vi "OCR_Build Lookup arrays.vi"(8 "Error":errorcluster) -> (0 "Error Out":errorcluster, 3 "Look Up Array Out":cluster{T1[]}[](array[cluster]))   [LabVIEW 2009]
doc: "Builds Lookup arrays from font list"
uses:
  Controls/Cluster/Cluster_Bit array and Character.ctl
  Controls/Array/Array Bool Char Bits Wide.ctl
  Controls/String_Picture/String Char Normal.ctl
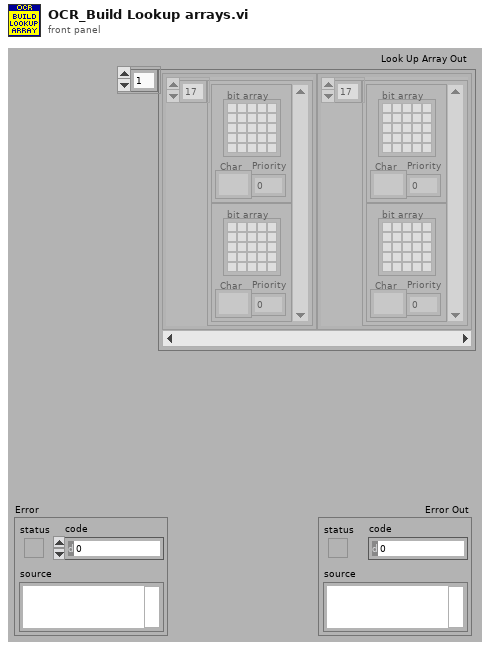
[diagram p1: front panel]
types:
  T1 = typedef "Cluster_Bit array and Character.ctl" = cluster{"bit array":T2, "Char":T3, "Priority":i32}
  T2 = typedef "Array Bool Char Bits Wide.ctl" = bool[][]
  T3 = typedef "String Char Normal.ctl" = string
  T4 = typedef "Cluster_Font Data.ctl" = cluster{"Font List Out":T5[], "Char Array":T3[], "Seperator Index":i32}
  T5 = typedef "Cluster_Character Data.ctl" = cluster{"Char":T3, "Wide":T2, "Med":T6, "Thin":T7, "Priority":i32}
  T6 = typedef "Array Bool Char Bits Med.ctl" = bool[][]
  T7 = typedef "Array Bool Char Bits Thin.ctl" = bool[][]
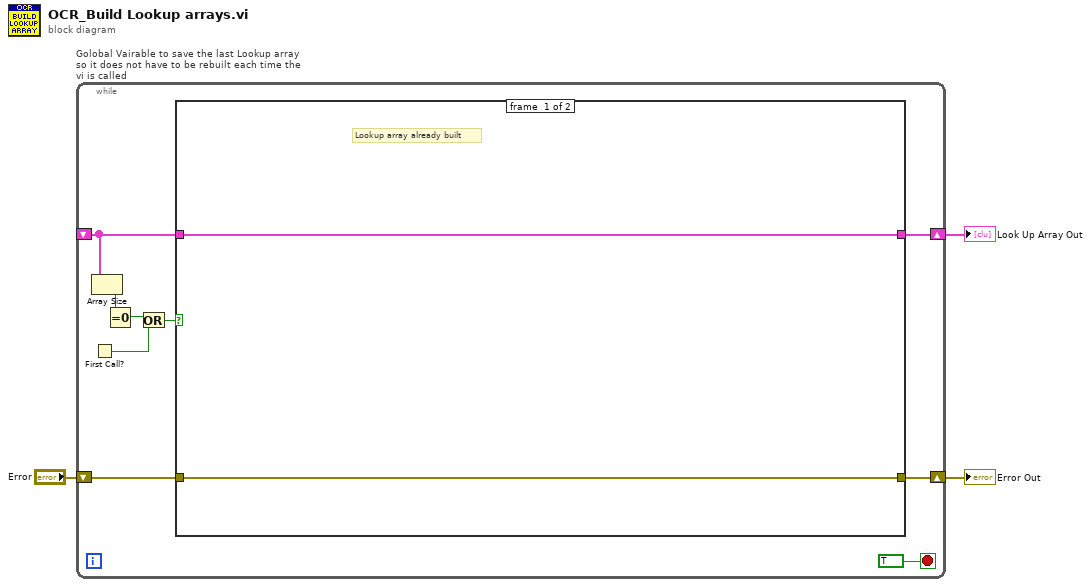
[diagram p0: block diagram]
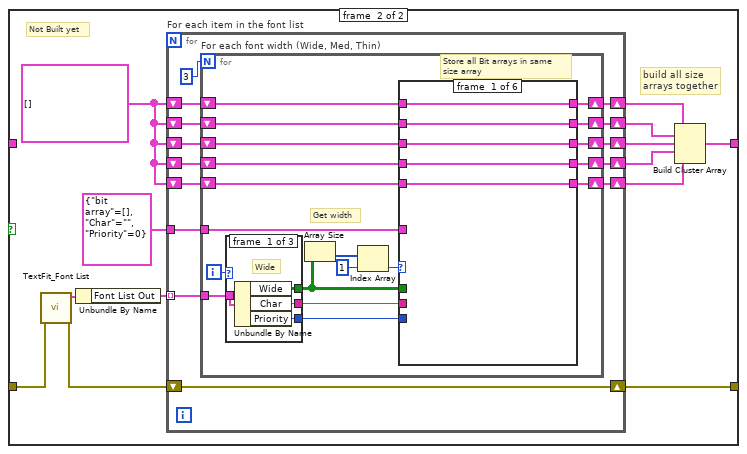
[diagram p2: hidden frame]
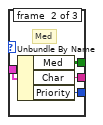
[diagram p3: hidden frame]
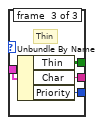
[diagram p4: hidden frame]
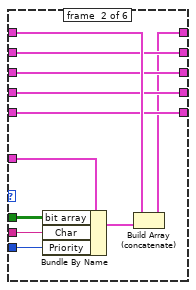
[diagram p5: hidden frame]
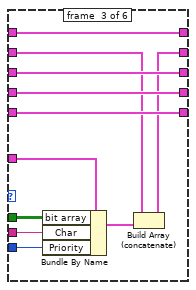
[diagram p6: hidden frame]
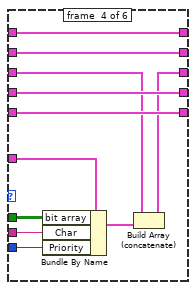
[diagram p7: hidden frame]
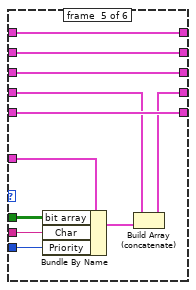
[diagram p8: hidden frame]
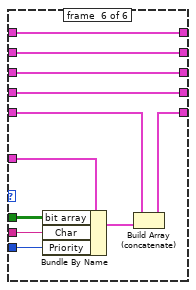
[diagram p9: hidden frame]
diagram:
  n1 = while "Golobal Vairable to save the last Lookup array so it does not have to be rebuilt each time the vi is called" {
    shift-right: [w11] -> w2
    shift-left: "Error" -> [w12]
    shift-right: [w10] -> w1
    shift-left: _ -> [w6]
    stop <- TRUE stop-if-true
    n2 = First Call?() -> (First Call?: T/F=w4:bool)
    n3 = Array Size(array=w6) -> (size(s)=w8:i32)
    n4 = Equal To 0?(x=w8) -> (x = 0?=w7:bool)
    n5 = Or(x=w7, y=w4) -> (x .or. y?=w5:bool)
    n6 = case shown="True" w5 {
      tunnel: w12 -> [w13 w27]
      tunnel: [w13 w26] -> w11
      tunnel: [w14 w15] -> w10
      tunnel: w6 -> [w14 _]
      frame #0 {
        # "Lookup array already built"
      }
      frame #1 {
        w22 = T1[] []
        # "build all size\narrays together"
        # "Not Built yet"
        n7 = call "TextFit_Font List.vi"("Error In"=w27) -> ("Error Out"=w25:errorcluster, "Font Cluster Out"=w24:T4)  [unwired: 9 in]
        n8 = Unbundle By Name(w24) -> ("Font List Out"=w23:T5[])
        n9 = for "For each item in the font list" {
          shift-right: [w41] -> w26
          shift-left: w25 -> [w41]
          tunnel: w23 -> [w38] mode=indexing
          shift-right: [w32] -> w19
          shift-left: w22 -> [w37]
          shift-right: [w31] -> w16
          shift-left: w22 -> [w36]
          shift-right: [w30] -> w20
          shift-left: w22 -> [w35]
          shift-right: [w29] -> w17
          shift-left: w22 -> [w34]
          shift-right: [w28] -> w18
          shift-left: w22 -> [w33]
          tunnel: T1 {"bit array"=[], "Char"="", "Priority"=0} ("bit char cluster") -> [w40]
          n10 = for "For each font width (Wide, Med, Thin)" {
            N: 3 -> [_]
            tunnel: w40 -> [w60]
            tunnel: w38 -> [w58]
            shift-right: [w43] -> w28
            shift-left: w33 -> [w48]
            shift-right: [w44] -> w29
            shift-left: w34 -> [w49]
            shift-right: [w45] -> w30
            shift-left: w35 -> [w50]
            shift-right: [w46] -> w31
            shift-left: w36 -> [w51]
            shift-right: [w47] -> w32
            shift-left: w37 -> [w52]
            i -> [w59]
            # "Store all Bit arrays in same\nsize array"
            # "Get width"
            n11 = case shown="..0" w59 {
              tunnel: w58 -> [w64 w68 w72]
              tunnel: [w63 w67 w71] -> w56
              tunnel: [w62 w66 w70] -> w57
              tunnel: [w61 w65 w69] -> w42
              frame #0 {
                # "Wide"
                n12 = Unbundle By Name(w64) -> ("Wide"=w63:T2, "Char"=w62:T3, "Priority"=w61:i32)
              }
              frame #1 {
                # "Med"
                n13 = Unbundle By Name(w68) -> ("Med"=w67:T6, "Char"=w66:T3, "Priority"=w65:i32)
              }
              frame #2 {
                # "Thin"
                n14 = Unbundle By Name(w72) -> ("Thin"=w71:T7, "Char"=w70:T3, "Priority"=w69:i32)
              }
            }
            n15 = Array Size(array=w56) -> (size(s)=w55:i32[])
            n16 = Index Array(array=w55, index=1) -> (element=w53:i32)
            n17 = case shown="3" w53 {
              tunnel: w60 -> [_ w83 w96 w108 w120 w132]
              tunnel: w56 -> [_ w81 w94 w106 w118 w130]
              tunnel: w57 -> [_ w82 w95 w107 w119 w131]
              tunnel: w52 -> [w77 w88 w92 w104 w116 w128]
              tunnel: w51 -> [w76 w87 w91 w101 w115 w127]
              tunnel: w50 -> [w75 w86 w99 w103 w112 w126]
              tunnel: w49 -> [w74 w85 w98 w110 w114 w123]
              tunnel: w48 -> [w73 w84 w97 w109 w121 w125]
              tunnel: [w77 w80 w92 w104 w116 w128] -> w47
              tunnel: [w76 w87 w90 w101 w115 w127] -> w46
              tunnel: [w75 w86 w99 w102 w112 w126] -> w45
              tunnel: [w74 w85 w98 w110 w113 w123] -> w44
              tunnel: [w73 w84 w97 w109 w121 w124] -> w43
              tunnel: w42 -> [_ w78 w89 w100 w111 w122]
              frame #0 {
              }
              frame #1 {
                n18 = Bundle By Name(cluster=w83, "bit array"=w81, "Char"=w82, "Priority"=w78) -> (w79:T1)
                n19 = Build Array (concatenate)(w88, w79) -> (w80:T1[])
              }
              frame #2 {
                n20 = Bundle By Name(cluster=w96, "bit array"=w94, "Char"=w95, "Priority"=w89) -> (w93:T1)
                n21 = Build Array (concatenate)(w91, w93) -> (w90:T1[])
              }
              frame #3 {
                n22 = Bundle By Name(cluster=w108, "bit array"=w106, "Char"=w107, "Priority"=w100) -> (w105:T1)
                n23 = Build Array (concatenate)(w103, w105) -> (w102:T1[])
              }
              frame #4 {
                n24 = Bundle By Name(cluster=w120, "bit array"=w118, "Char"=w119, "Priority"=w111) -> (w117:T1)
                n25 = Build Array (concatenate)(w114, w117) -> (w113:T1[])
              }
              frame #5 {
                n26 = Bundle By Name(cluster=w132, "bit array"=w130, "Char"=w131, "Priority"=w122) -> (w129:T1)
                n27 = Build Array (concatenate)(w125, w129) -> (w124:T1[])
              }
            }
          }
        }
        n28 = Build Cluster Array(w19, w16, w20, w17, w18) -> (w15:cluster{T1[]}[])
      }
    }
  }
  "Error Out" <- w2
  "Look Up Array Out" <- w1
